vi "logging_set.vi"(8 "error in":errorcluster, 10 "Logging target":string, 11 "VISA resource name":refnum<visa-resource-name>) -> (0 "error out":errorcluster, 3 "VISA resource name out":refnum<visa-resource-name>)   [LabVIEW 2014, in "rszvl_rsidr_core.lvlib"]
uses:
  rszvl_rsidr_core.lvlib
  type_Logging_Parameter.ctl
  type_Error_Codes.ctl
  Match Regular Expression.xnode
panel:
  # "Supported formats:\nUDP:<Local_Port>:<Remote_Port>:<Remote_Host>\n         e.g. UDP:61556:61557:localhost -alias=\nFILE:0-new/1-add:<path>"
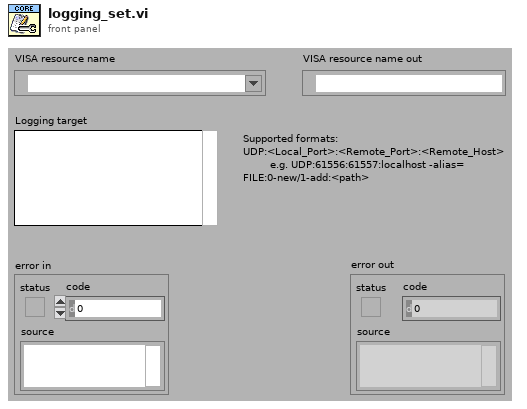
[diagram p1: front panel]
types:
  T1 = typedef "rszvl_rsidr_core.lvlib/type_Logging_Parameter.ctl" = enum16{"Type (String)", "SessionAlias(String)", "FormatString (String)", "UDPconectionID (I32)", "UDPlocalPort (I32)", "UDPremotePort (I32)", "UDPremoteHost (String)", "FILEmode (I32)", "FILEpath (String)", "FILEopenID (I32)"}
  T2 = enum16{"open", "replace", "create", "open or create", "replace or create", "replace or create with confirmation"}
  T3 = typedef "rszvl_rsidr_core.lvlib/type_Error_Codes.ctl" = enum16{"No_error", "VISA_err_ResourceNotFound", "VISA_err_Timeout", "VISA_warn_MoreDataAvailable", "RS_err_MissingCallback", "RS_err_InvalidAttribute", "RS_err_InvalidValue", "RS_err_UnknownResource", "RS_err_AlreadyInitialized", "RS_err_InstrumentStatus", "RS_err_BadRepCapName", "RS_err_TypesMismatch", "RS_err_ValueNotSupported", "RS_err_InvalidRngTable", "RS_err_IDqueryFail", "RS_err_UnexpResponse", "VISA_warn_ConfigNotLoaded", "RS_err_AttributeNotReadable", "RS_err_AttributeNotWritable", "RS_err_InstrumentType", "RS_err_InstrumentOption", "VISA_err_InvalidSize", "RS_err_ReliabilityIndicator", "VISA_warn_UnknownStatus", "VISA_warn_TermCharRead", "VISA_err_IO_error"}
  T4 = typedef "rszvl_rsidr_core.lvlib/type_Session_Data.ctl" = cluster{"Instr type":string, "Instr type for err. msg.":string, "Installed Options":string[], "OPC Timeout":i32, "Query Instrument Status":bool, "Check Range":bool, "Check Options":bool, "Add LF to Write":bool, "Simulate":bool, "Logging":bool, "Logging params":variant, "Interface Type":enum16{"Unknown", "GPIB", "VXI", "GPIB_VXI", "ASRL", "PXI", "TCPIP", "USB", "SOCKET"}, "Fast Sweep":i32, "AdditionalFlags":i32, "WaitBeforeWrite":i32, "WaitBeforeRead":i32, "BinDataChunkSize":i64}
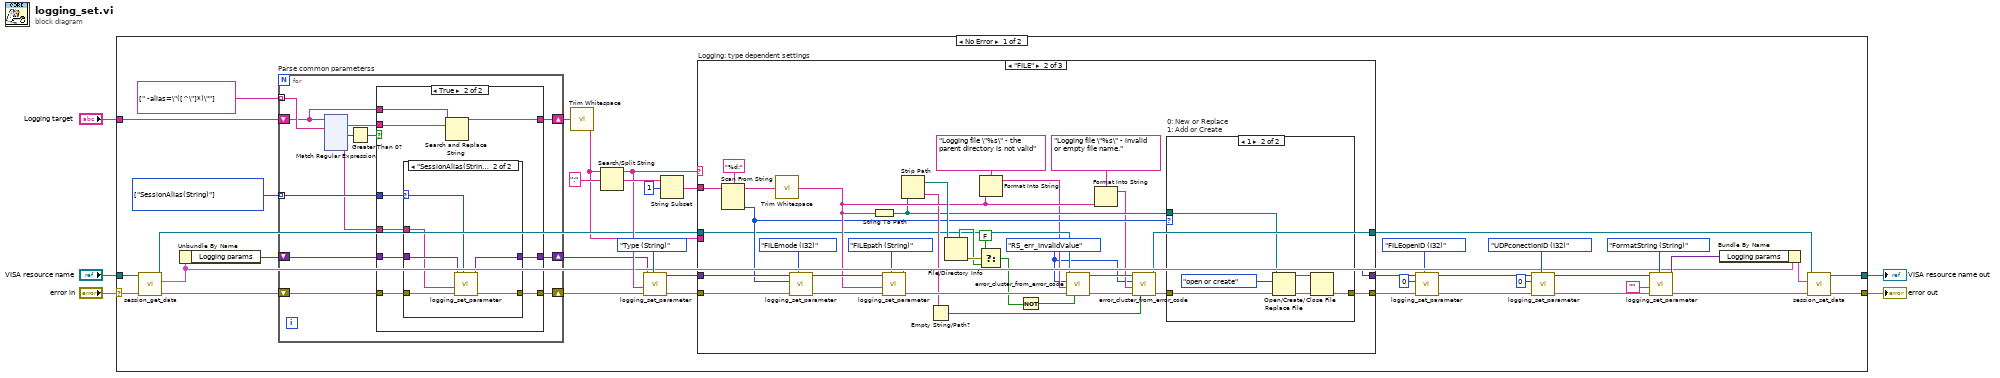
[diagram p0: block diagram]
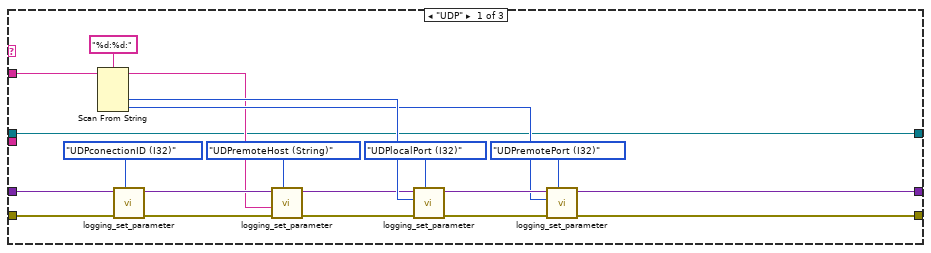
[diagram p4: hidden frame]
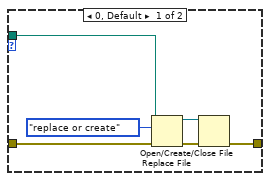
[diagram p5: hidden frame]
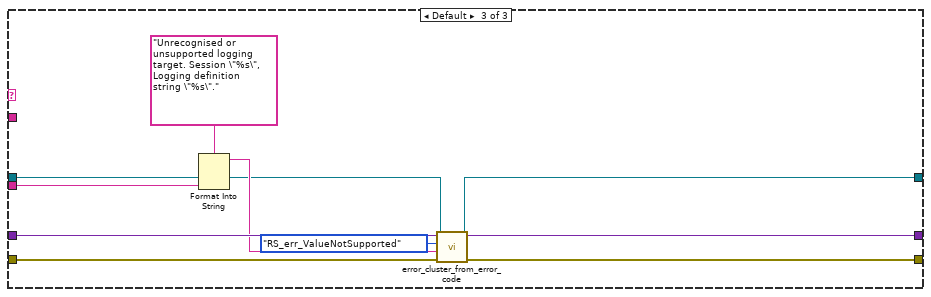
[diagram p6: hidden frame]
diagram:
  n1 = case shown="No Error" "error in" {
    selector: "error in" -> [w40 w265]
    tunnel: [w39 w265] -> w2
    tunnel: "VISA resource name" -> [w12 w264]
    tunnel: "Logging target" -> [w16 _]
    tunnel: [w38 w264] -> w1
    frame No Error {
      w9 = T1[] [enum."SessionAlias(String)"] items=["Type (String)", "SessionAlias(String)", "FormatString (String)", "UDPconectionID (I32)", "UDPlocalPort (I32)", "UDPremotePort (I32)", "UDPremoteHost (String)", "FILEmode (I32)", "FILEpath (String)", "FILEopenID (I32)"]
      n2 = call "session_get_data.vi"("error in"=w40, "VISA resource name"=w12) -> ("error out"=w8:errorcluster, "Session User Data out"=w27:T4, "VISA resource name out"=w25:refnum<visa-resource-name>)  [unwired: 7 in]
      n3 = Unbundle By Name(w27) -> ("Logging params"=w11:variant)
      n4 = for "Parse common parameterss" {
        shift-right: [w51] -> w14
        shift-left: w16 -> [w52]
        tunnel: string[] [" -alias=\"([^\"]*)\""] -> [w56] mode=indexing
        shift-right: [w46] -> w10
        shift-left: w11 -> [w50]
        tunnel: w9 -> [w49] mode=indexing
        shift-right: [w45] -> w7
        shift-left: w8 -> [w48]
        n5 = xnode ("Match Regular Expression")("input string"=w52, "regular expression"=w56) -> ("whole match"=w53:string, "offset past match"=w55:i32, "submatch 1"=w47:string)  [unwired: 4 in, 3 out]
        n6 = Greater Than 0?(x=w55) -> (x > 0?=w54:bool)
        n7 = case shown="True" w54 {
          tunnel: w53 -> [_ w66]
          tunnel: w52 -> [w59 w67]
          tunnel: [w59 w68] -> w51
          tunnel: w50 -> [w58 w63]
          tunnel: w47 -> [_ w61]
          tunnel: w49 -> [_ w64]
          tunnel: w48 -> [w57 w65]
          tunnel: [w58 w62] -> w46
          tunnel: [w57 w60] -> w45
          frame False {
          }
          frame True {
            n8 = case shown="\"SessionAlias(String)\"" w64 {
              selector: w64 -> [_ w73]
              tunnel: w65 -> [w69 w76]
              tunnel: w63 -> [w70 w75]
              tunnel: [w70 w74] -> w62
              tunnel: w61 -> [_ w72]
              tunnel: [w69 w71] -> w60
              frame Default {
              }
              frame "SessionAlias(String)" {
                n9 = call "logging_set_parameter.vi"("Logging Parameter"=w73, "error in"=w76, "String parameter (\"\")"=w72, "Logging params in"=w75) -> ("error out"=w71:errorcluster, "Logging params out"=w74:variant)  [unwired: 6 in]
              }
            }
            n10 = Search and Replace String(input string=w67, search string=w66) -> (result string=w68:string)  [unwired: 6 in, 3 out]
          }
        }
      }
      n11 = call "Trim Whitespace.vi"("string"=w14) -> ("trimmed string"=w13:string)  [unwired: 1 in]
      n12 = Search/Split String(string=w13, search string/char (-)=":") -> (substring before match=w34:string, match + rest of string=w43:string)  [unwired: 1 in, 1 out]
      n13 = call "logging_set_parameter.vi"("Logging Parameter"=type_Logging_Parameter."Type (String)", "error in"=w7, "String parameter (\"\")"=w34, "Logging params in"=w10) -> ("error out"=w36:errorcluster, "Logging params out"=w35:variant)  [unwired: 6 in]
      n14 = String Subset(string=w43, offset (0)=1) -> (substring=w41:string)  [unwired: 1 in]
      n15 = case "Logging: type dependent settings" shown="\"FILE\"" w34 {
        tunnel: w36 -> [w208 w238 w260]
        tunnel: w41 -> [w209 w242 _]
        tunnel: w35 -> [w193 w239 w259]
        tunnel: [w207 w216 w263] -> w20
        tunnel: w13 -> [_ _ w262]
        tunnel: w25 -> [w190 w215 w256]
        tunnel: [w192 w220 w259] -> w18
        tunnel: [w190 w213 w255] -> w6
        frame "UDP" {
          n16 = Scan From String(format string="%d:%d:", input string=w209) -> (remaining string=w191:string, output 1=w200:i32, output 2=w194:i32)  [unwired: 4 in, 2 out]
          n17 = call "logging_set_parameter.vi"("Logging Parameter"=type_Logging_Parameter."UDPconectionID (I32)", "error in"=w208, "Logging params in"=w193) -> ("error out"=w203:errorcluster, "Logging params out"=w202:variant)  [unwired: 7 in]
          n18 = call "logging_set_parameter.vi"("Logging Parameter"=type_Logging_Parameter."UDPremoteHost (String)", "error in"=w203, "String parameter (\"\")"=w191, "Logging params in"=w202) -> ("error out"=w198:errorcluster, "Logging params out"=w195:variant)  [unwired: 6 in]
          n19 = call "logging_set_parameter.vi"("Logging Parameter"=type_Logging_Parameter."UDPlocalPort (I32)", "error in"=w198, "I32 parameter (0)"=w200, "Logging params in"=w195) -> ("error out"=w197:errorcluster, "Logging params out"=w196:variant)  [unwired: 6 in]
          n20 = call "logging_set_parameter.vi"("Logging Parameter"=type_Logging_Parameter."UDPremotePort (I32)", "error in"=w197, "I32 parameter (0)"=w194, "Logging params in"=w196) -> ("error out"=w207:errorcluster, "Logging params out"=w192:variant)  [unwired: 6 in]
        }
        frame "FILE" {
          w210 = type_Error_Codes."RS_err_InvalidValue" ("Error Enum in")
          n21 = Scan From String(format string="%d:", input string=w242) -> (remaining string=w224:string, output 1=w219:i32)  [unwired: 3 in, 2 out]
          n22 = call "Trim Whitespace.vi"("string"=w224) -> ("trimmed string"=w223:string)  [unwired: 1 in]
          n23 = call "logging_set_parameter.vi"("Logging Parameter"=type_Logging_Parameter."FILEmode (I32)", "error in"=w238, "I32 parameter (0)"=w219, "Logging params in"=w239) -> ("error out"=w237:errorcluster, "Logging params out"=w235:variant)  [unwired: 6 in]
          n24 = String To Path(string=w223) -> (path=w217:path)
          n25 = call "logging_set_parameter.vi"("Logging Parameter"=type_Logging_Parameter."FILEpath (String)", "error in"=w237, "String parameter (\"\")"=w223, "Logging params in"=w235) -> ("error out"=w234:errorcluster, "Logging params out"=w220:variant)  [unwired: 6 in]
          n26 = Strip Path(path=w217) -> (stripped path=w225:path, name=w221:string)
          n27 = Empty String/Path?(string/path=w221) -> (empty?=w222:bool)
          n28 = File/Directory Info(path=w225) -> (directory=w232:bool, error out=w233:errorcluster)  [unwired: 1 in, 5 out]
          n29 = Format Into String(format string="Logging file \"%s\" - the parent directory is not valid", w223) -> (resulting string=w211:string)  [unwired: 2 in, 1 out]
          n30 = Select(t=FALSE, s=w233, f=w232) -> (s? t:f=w230:bool)
          n31 = Not(x=w230) -> (.not. x?=w229:bool)
          n32 = call "error_cluster_from_error_code.vi"("error creation enabled (T)"=w229, "error in"=w234, "error message (\"\")"=w211, "Error Enum in"=w210, "VISA resource name"=w215) -> ("error out"=w227:errorcluster, "VISA resource name out"=w214:refnum<visa-resource-name>)  [unwired: 5 in]
          n33 = Format Into String(format string="Logging file \"%s\" - invalid or empty file name.", w223) -> (resulting string=w212:string)  [unwired: 2 in, 1 out]
          n34 = call "error_cluster_from_error_code.vi"("error creation enabled (T)"=w222, "error in"=w227, "error message (\"\")"=w212, "Error Enum in"=w210, "VISA resource name"=w214) -> ("error out"=w218:errorcluster, "VISA resource name out"=w213:refnum<visa-resource-name>)  [unwired: 5 in]
          n35 = case "0: New or Replace\n1: Add or Create" shown="1" w219 {
            tunnel: w218 -> [w248 w254]
            tunnel: w217 -> [w247 w253]
            tunnel: [w243 w249] -> w216
            frame 0, Default {
              n36 = Open/Create/Replace File(file path (use dialog)=w247, error in=w248, operation (0:open)=T2."replace or create") -> (refnum out=w244:refnum<file>, error out=w245:errorcluster)  [unwired: 3 in, 1 out]
              n37 = Close File(refnum=w244, error in=w245) -> (error out=w243:errorcluster)  [unwired: 1 out]
            }
            frame 1 {
              n38 = Open/Create/Replace File(file path (use dialog)=w253, error in=w254, operation (0:open)=T2."open or create") -> (refnum out=w250:refnum<file>, error out=w251:errorcluster)  [unwired: 3 in, 1 out]
              n39 = Close File(refnum=w250, error in=w251) -> (error out=w249:errorcluster)  [unwired: 1 out]
            }
          }
        }
        frame Default {
          n40 = Format Into String(format string="Unrecognised or unsupported logging target. Session \"%s\", Logging definition string \"%s\".", w256, w262) -> (resulting string=w258:string)  [unwired: 2 in, 1 out]
          n41 = call "error_cluster_from_error_code.vi"("error in"=w260, "error message (\"\")"=w258, "Error Enum in"=type_Error_Codes."RS_err_ValueNotSupported", "VISA resource name"=w256) -> ("error out"=w263:errorcluster, "VISA resource name out"=w255:refnum<visa-resource-name>)  [unwired: 6 in]
        }
      }
      n42 = call "logging_set_parameter.vi"("Logging Parameter"=type_Logging_Parameter."FILEopenID (I32)", "error in"=w20, "I32 parameter (0)"=0, "Logging params in"=w18) -> ("error out"=w19:errorcluster, "Logging params out"=w17:variant)  [unwired: 6 in]
      n43 = call "logging_set_parameter.vi"("Logging Parameter"=type_Logging_Parameter."UDPconectionID (I32)", "error in"=w19, "I32 parameter (0)"=0, "Logging params in"=w17) -> ("error out"=w31:errorcluster, "Logging params out"=w29:variant)  [unwired: 6 in]
      n44 = call "logging_set_parameter.vi"("Logging Parameter"=type_Logging_Parameter."FormatString (String)", "error in"=w31, "String parameter (\"\")"="" ("Empty String Constant"), "Logging params in"=w29) -> ("error out"=w30:errorcluster, "Logging params out"=w28:variant)  [unwired: 6 in]
      n45 = Bundle By Name(cluster=w27, "Logging params"=w28) -> (w26:T4)
      n46 = call "session_set_data.vi"("error in"=w30, "Session User Data in"=w26, "VISA resource name"=w6) -> ("error out"=w39:errorcluster, "VISA resource name out"=w38:refnum<visa-resource-name>)  [unwired: 7 in]
    }
    frame Error {
    }
  }
  "VISA resource name out" <- w1
  "error out" <- w2
